vi "Report Firmware.vi"(6 "Queue Name":string="firmata-serial-communication", 8 "error in (no error)":errorcluster) -> (0 "error out":errorcluster, 2 "FirmataFirmwareVersion":string, 3 "FirmataFirmwareName":string)   [LabVIEW 2020, in "FirmataClient.lvlib"]
doc: "Request the firmware name and version running on the target board."
uses:
  FirmataClient.lvlib
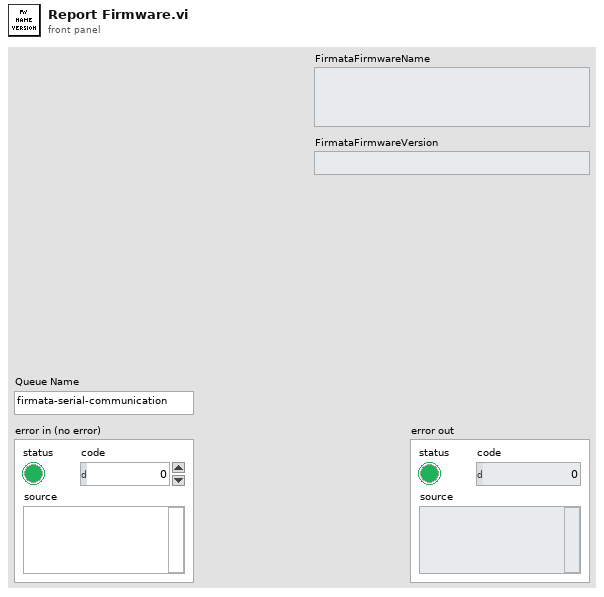
[diagram p1: front panel]
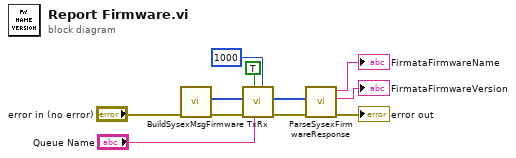
[diagram p0: block diagram]
diagram:
  n1 = call "BuildSysexMsgFirmware.vi"("error in"="error in (no error)") -> ("error out"=w7:errorcluster, "GetFirmwareMessage"=w5:u8[])  [unwired: 7 in, 2 out]
  n2 = call "TxRx.vi"("Reply Timeout Ms"=1000, "Queue Name"="Queue Name", "Wait For Reply?"=TRUE, "error in"=w7, "Message"=w5) -> ("error out"=w6:errorcluster, "Reply"=w4:u8[])  [unwired: 5 in]
  n3 = call "ParseSysexFirmwareResponse.vi"("error in"=w6, "Sysex Message"=w4) -> ("error out"=→"error out":errorcluster, "FirmataFirmwareVersion"=→"FirmataFirmwareVersion":string, "FirmataFirmwareName"=→"FirmataFirmwareName":string)  [unwired: 6 in, 1 out]
